vi "X_2.57_tabcontroll.vi"() -> ()   [LabVIEW 2022 SP3]
uses:
  <vilib>/numeric/Random Number (Range) DBL.vi
panel:
  in  "Tab Control":enum32{"Input", "Graf", "Data"}(tab)
  in  "Ventetid imellem iteration":dbl=100.0 min=50.0 max=500.0
  in  "Øvre granse":dbl=100.0 min=2.0
  in  "Nedre granse":dbl=1.0 min=1.0 max=99.0
  in  "Start tab":enum16{"Input", "Graf", "Data"}(ring)
  in  "stop":bool
  in  "stop 2":bool
  out "Waveform Chart":dbl(graph)
  out "Iterationer":dbl
  in  "stop 3":bool
  out "Mean":dbl
  out "Spredning":dbl
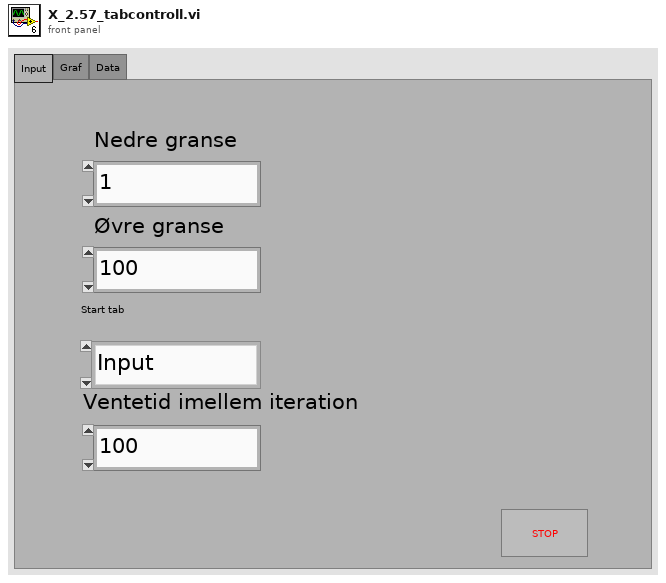
[diagram p1: front panel]
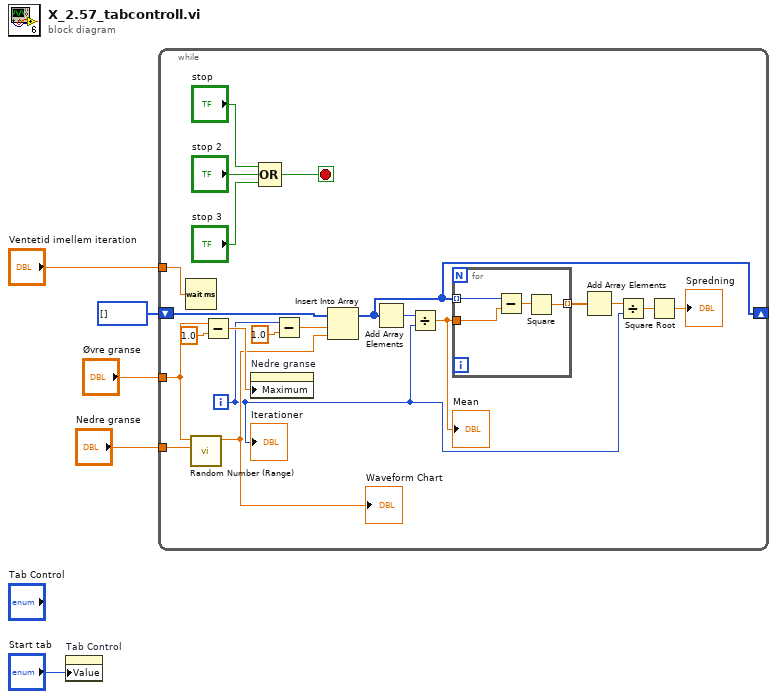
[diagram p0: block diagram]
diagram:
  n1 = property on="Tab Control" class="TabCtl (strict)"("Value"="Start tab") -> ()  [unwired: 2 in, 2 out]
  n2 = while {
    tunnel: "Øvre granse" -> [w24]
    tunnel: "Nedre granse" -> [w23]
    tunnel: "Ventetid imellem iteration" -> [w22]
    shift-right: [w12] -> _
    shift-left: i32[] [] -> [w16]
    i -> [w8]
    stop <- w18 stop-if-true
    n3 = Wait (ms)(milliseconds to wait=w22) -> ()  [unwired: 1 out]
    n4 = call-poly <vilib>:"Random Number (Range).vi"("lower bound (0)"=w23, "upper bound (100)"=w24) -> ("number"=w17:dbl)  [unwired: 9 in]
    "Waveform Chart" <- w17
    n5 = Subtract(x=w24, y=1.0) -> (x-y=w25:dbl)
    n6 = property on="Nedre granse" class="DigNum (strict)"("Maximum"=w25) -> ()  [unwired: 2 in, 2 out]
    n7 = Compound Arithmetic op=OR("stop", "stop 2", "stop 3") -> (w18:bool)
    n8 = Subtract(x=w8, y=1.0) -> (x-y=w13:dbl)
    n9 = Insert Into Array(array=w16, index=w13, new element=w17) -> (w12:i32[])
    n10 = Add Array Elements(numeric array=w12) -> (sum=w14:i32)
    n11 = Divide(x=w14, y=w8) -> (x/y=w11:dbl)
    "Mean" <- w11
    n12 = for {
      tunnel: w12 -> [w30] mode=indexing
      tunnel: w11 -> [w29]
      tunnel: [w27] -> w10 mode=indexing
      n13 = Subtract(x=w30, y=w29) -> (x-y=w28:dbl)
      n14 = Square(x=w28) -> (x^2=w27:dbl)
    }
    n15 = Add Array Elements(numeric array=w10) -> (sum=w9:dbl)
    n16 = Divide(x=w9, y=w8) -> (x/y=w7:dbl)
    n17 = Square Root(x=w7) -> (sqrt(x)=→"Spredning":dbl)
    "Iterationer" <- w8
  }
